vi "Main-20220212.vi"   [LabVIEW 2019]
uses:
  ctl/move.ctl
  ctl/continued move array-V2.ctl
types:
  T1 = typedef "continued move array-V2.ctl" = cluster{"X":dbl, "Y":dbl, "Speed":dbl, "rotate\ndegree":dbl, "deg":dbl}
  T2 = typedef "move.ctl" = enum16{"S - box", "box - R1", "R1 - box", "box - R2", "R2 - box", "box - R3", "R3 - box", "box - R4", "R4 - box", "box - R5", "R5 - box", "box - rec", "rec - box", "box - S", "box align", "box end"}
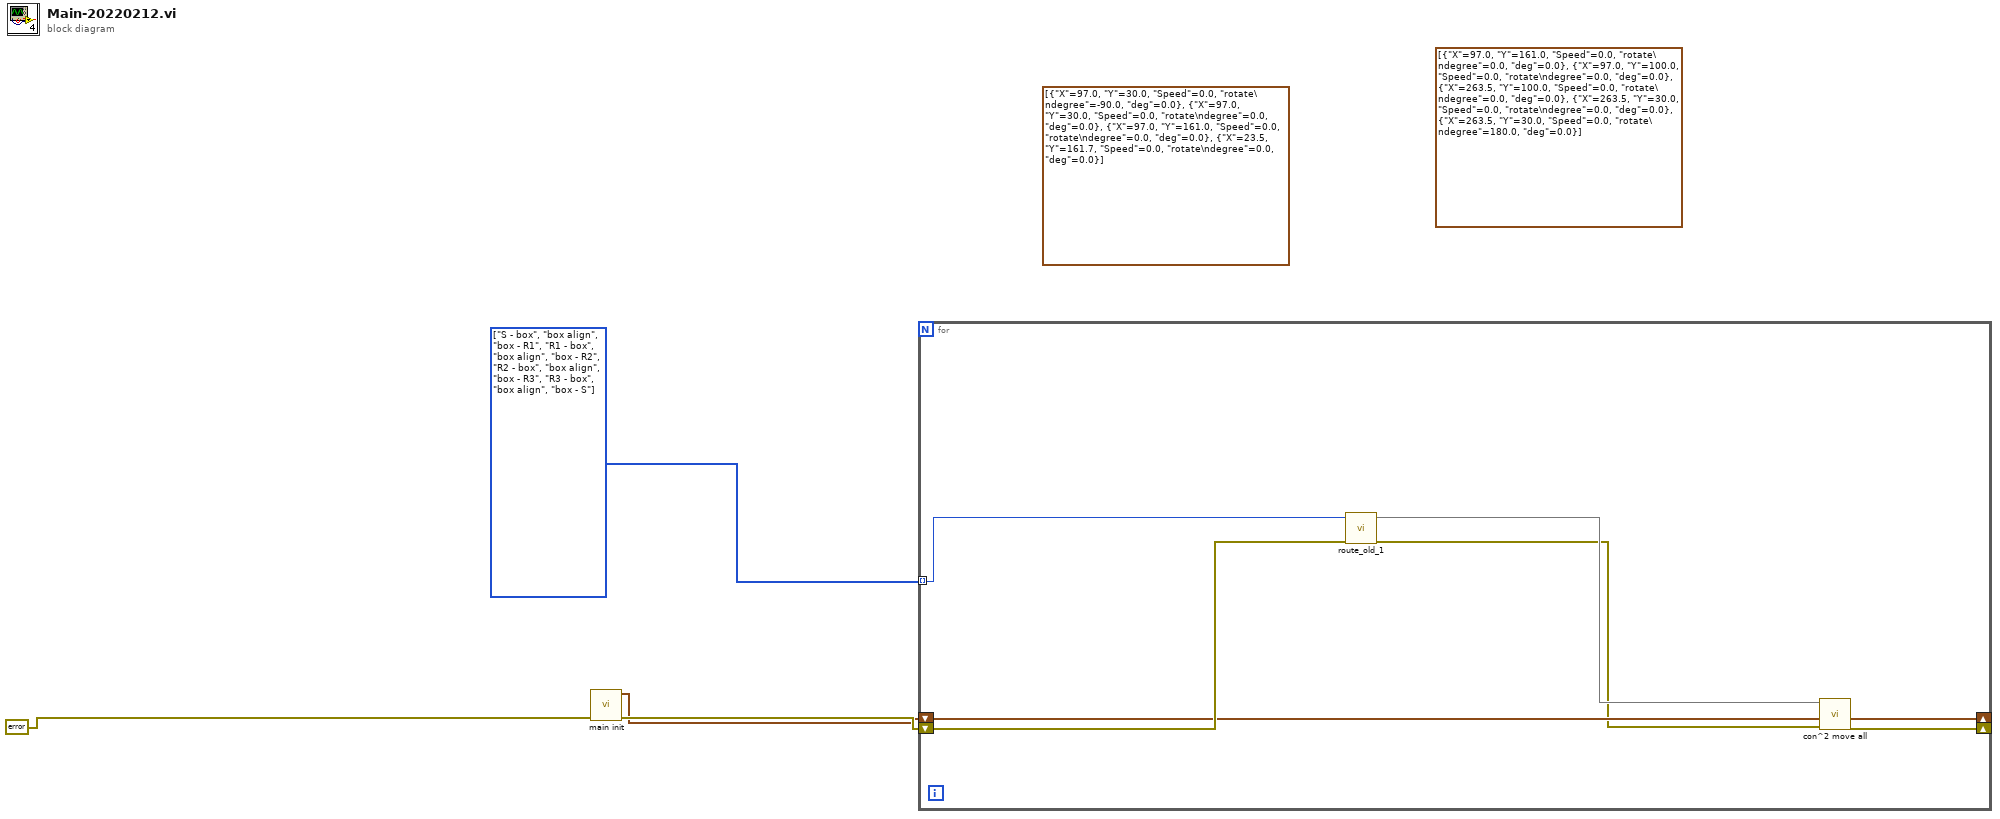
[diagram p0: block diagram]
diagram:
  (unwired) T1[] [{"X"=97.0, "Y"=161.0, "Speed"=0.0, "rotate\ndegree"=0.0, "deg"=0.0}, {"X"=97.0, "Y"=100.0, "Speed"=0.0, "rotate\ndegree"=0.0, "deg"=0.0}, {"X"=263.5, "Y"=100.0, "Speed"=0.0, "rotate\ndegree"=0.0, "deg"=0.0}, {"X"=263.5, "Y"=30.0, "Speed"=0.0, "rotate\ndegree"=0.0, "deg"=0.0}, {"X"=263.5, "Y"=30.0, "Speed"=0.0, "rotate\ndegree"=180.0, "deg"=0.0}] ("contrast move array")
  (unwired) T1[] [{"X"=97.0, "Y"=30.0, "Speed"=0.0, "rotate\ndegree"=-90.0, "deg"=0.0}, {"X"=97.0, "Y"=30.0, "Speed"=0.0, "rotate\ndegree"=0.0, "deg"=0.0}, {"X"=97.0, "Y"=161.0, "Speed"=0.0, "rotate\ndegree"=0.0, "deg"=0.0}, {"X"=23.5, "Y"=161.7, "Speed"=0.0, "rotate\ndegree"=0.0, "deg"=0.0}] ("contrast move array")
  w4 = T2[] [enum."S - box", enum."box align", enum."box - R1", enum."R1 - box", enum."box align", enum."box - R2", enum."R2 - box", enum."box align", enum."box - R3", enum."R3 - box", enum."box align", enum."box - S"] items=["S - box", "box - R1", "R1 - box", "box - R2", "R2 - box", "box - R3", "R3 - box", "box - R4", "R4 - box", "box - R5", "R5 - box", "box - rec", "rec - box", "box - S", "box align", "box end"]
  n1 = call "main init.vi"("error in (no error)"=errorcluster {"status"=FALSE, "code"=0, "source"=""} ("error out")) -> ("error out"=w3:errorcluster, "position out"=w2:cluster{"x":dbl, "y":dbl, "degree":dbl})  [unwired: 9 in]
  n2 = for {
    tunnel: w4 -> [w11] mode=indexing
    shift-right: [w9] -> _
    shift-left: w2 -> [w7]
    shift-right: [w6] -> _
    shift-left: w3 -> [w8]
    n3 = call "route_old_1.vi"("error in (no error)"=w8, "Enum"=w11) -> ("error out"=w5:errorcluster, 3:w10)  [unwired: 7 in, 1 out]
    n4 = call "con^2 move all.vi"("error in (no error)"=w5, "now position"=w7, "contrast move array"=w10) -> ("error out"=w6:errorcluster, "position out"=w9:cluster{"x":dbl, "y":dbl, "degree":dbl})  [unwired: 7 in]
  }
